vi "Get Account Info.vi"(8 "error in (no error)":errorcluster, 10 "Account Number":string, 11 "Accounts info":T1) -> (0 "error out":errorcluster, 2 "Valid Account?":bool, 3 "Account Info":T2, 5 "Index of Account":i32)   [LabVIEW 2020, in "ATM.lvlib"]
doc: "Once the Account is inserted, this VI search for the account info, in case doesn't exist, returns a False Flag"
uses:
  ATM.lvlib
  Account Info -- cluster.ctl
  Accounts Info -- cluster.ctl
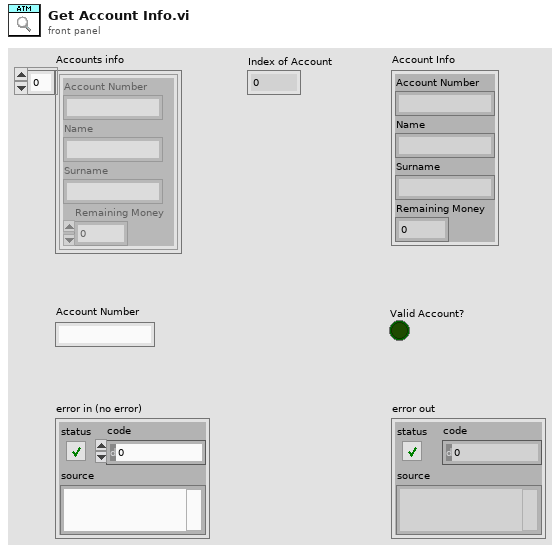
[diagram p1: front panel]
types:
  T1 = typedef "ATM.lvlib/Accounts Info -- cluster.ctl" = T2[]
  T2 = typedef "ATM.lvlib/Account Info -- cluster.ctl" = cluster{"Account Number":string, "Name":string, "Surname":string, "Remaining Money":i32}
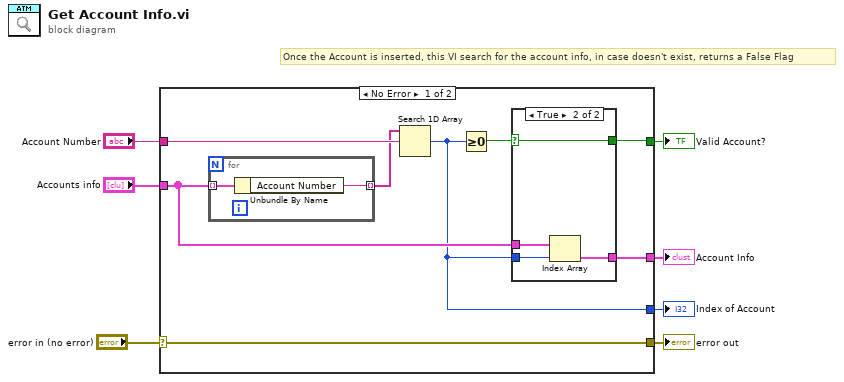
[diagram p0: block diagram]
diagram:
  # "Once the Account is inserted, this VI search for the account info, in case doesn't exist, returns a False Flag"
  n1 = case shown="No Error" "error in (no error)" {
    selector: "error in (no error)" -> [w11 w23]
    tunnel: [w14 _] -> w7
    tunnel: "Account Number" -> [w15 _]
    tunnel: [w11 w23] -> w4
    tunnel: [w9 _] -> w3
    tunnel: "Accounts info" -> [w10 _]
    tunnel: [w8 _] -> w1
    frame No Error {
      n2 = for {
        tunnel: [w22] -> w12 mode=indexing
        tunnel: w10 -> [w21] mode=indexing
        n3 = Unbundle By Name(w21) -> ("Account Number"=w22:string)
      }
      n4 = Search 1D Array(1D array=w12, element=w15) -> (index of element=w8:i32)  [unwired: 1 in]
      n5 = Greater Or Equal To 0?(x=w8) -> (x >= 0?=w13:bool)
      n6 = case shown="True" w13 {
        selector: w13 -> [w16 w20]
        tunnel: [w16 w20] -> w14
        tunnel: w10 -> [_ w19]
        tunnel: w8 -> [_ w18]
        tunnel: [_ w17] -> w9
        frame False {
        }
        frame True {
          n7 = Index Array(array=w19, index=w18) -> (element=w17:T2)
        }
      }
    }
    frame Error {
    }
  }
  "Valid Account?" <- w7
  "error out" <- w4
  "Account Info" <- w3
  "Index of Account" <- w1
